vi "E441X_PM_Get_Status_Registers.vi"(0 "VISA session":refnum<visa-resource-name>, 5 "Register (4: Questionable Status Register)":i32(ring)=4 items=["Service Request Enable Register (SRE)", "Standard Event Status Enable Register (ESE)", "Device Status Register", "Operation Status Register", "Questionable Status Register", "Operation Status Calibration", "Operation Status Measuring", "Operation Status Trigger", "Operation Status Sense", "Operation Status Low Limit Fail", "Operation Status Upper Limit Fail", "Questionable Status Power", "Questionable Status Calibration"], 7 "Register Part (2: Enable)":i32(ring)=2 items=["Enable"=2, "Negative Transition"=0, "Positive Transition"=1, "Event"=3, "Condition"=4], 11 "error in (no error)":errorcluster {"code" format="%.0x"}) -> (4 "dup VISA session":refnum<visa-resource-name>, 10 "State":u16, 15 "error out":errorcluster {"code" format="%.0x"})   [LabVIEW 2015]
doc: "This VI returns the instrument status registers state."
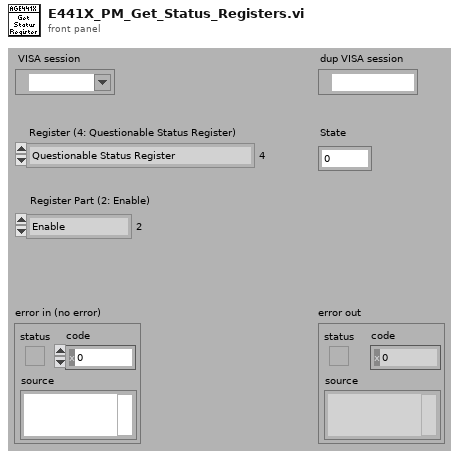
[diagram p1: front panel]
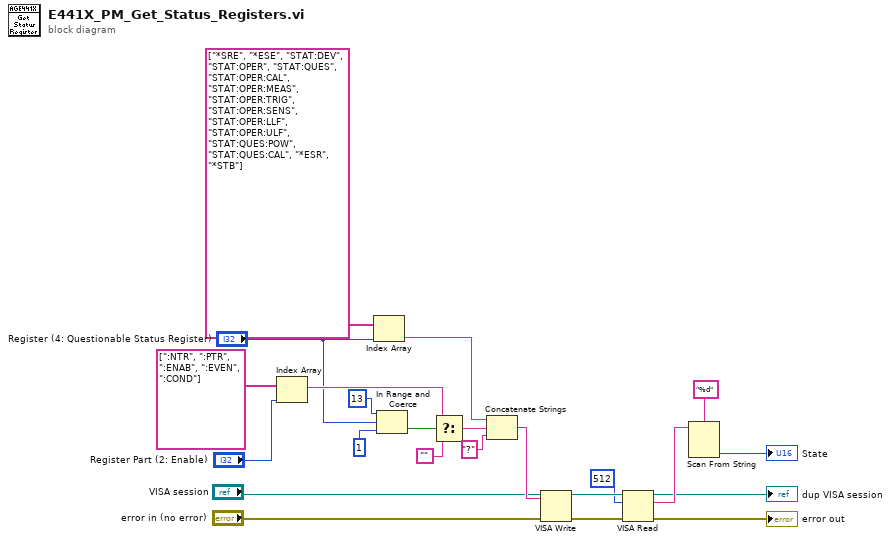
[diagram p0: block diagram]
diagram:
  n1 = Index Array(array=string[] [":NTR", ":PTR", ":ENAB", ":EVEN", ":COND"], index="Register Part (2: Enable)") -> (element=w23:string)
  n2 = Index Array(array=string[] ["*SRE", "*ESE", "STAT:DEV", "STAT:OPER", "STAT:QUES", "STAT:OPER:CAL", "STAT:OPER:MEAS", "STAT:OPER:TRIG", "STAT:OPER:SENS", "STAT:OPER:LLF", "STAT:OPER:ULF", "STAT:QUES:POW", "STAT:QUES:CAL", "*ESR", "*STB"], index="Register (4: Questionable Status Register)") -> (element=w22:string)
  n3 = In Range and Coerce(upper limit=13, x="Register (4: Questionable Status Register)", lower limit=1 ("y")) -> (In Range?=w14:bool)  [unwired: 1 out]
  n4 = Select(t=w23, s=w14, f="") -> (s? t:f=w21:string)
  n5 = Concatenate Strings(w22, w21, "?" ("string")) -> (w20:string)
  n6 = VISA Write(VISA resource name="VISA session", write buffer=w20, error in (no error)="error in (no error)") -> (VISA resource name out=w8:refnum<visa-resource-name>, error out=w7:errorcluster)  [unwired: 1 out]
  n7 = VISA Read(VISA resource name=w8, byte count=u32 512 ("byte count (0)"), error in (no error)=w7) -> (VISA resource name out=→"dup VISA session":refnum<visa-resource-name>, read buffer=w5:string, error out=→"error out":errorcluster)  [unwired: 1 out]
  n8 = Scan From String(format string="%d", input string=w5) -> (output 1=→"State":u16)  [unwired: 3 in, 3 out]
